vi "Write Assert Name List.vi"(10 "Assert Name List":variant, 11 "Base Display Configuration in":refnum<class "Base Display Configuration.lvclass">) -> (3 "Base Display Configuration out":refnum<class "Base Display Configuration.lvclass">)   [LabVIEW 2016, in "Assert API Components.lvlib" / "Assert Display.lvlib" / "Main Display.lvlib" / "Base Display Configuration.lvclass"]
uses:
  Base Display Configuration.lvclass
  Base Display Configuration.lvclass/Base Display Configuration.ctl
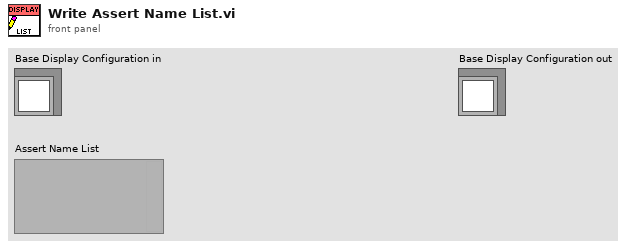
[diagram p1: front panel]
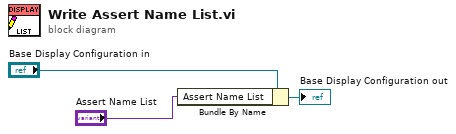
[diagram p0: block diagram]
diagram:
  n1 = Bundle By Name(cluster="Base Display Configuration in", "Assert Name List"="Assert Name List") -> (→"Base Display Configuration out":refnum<class "Base Display Configuration.lvclass">)
